vi "Read Theme.vi"(8 "error in":errorcluster, 11 "Theme in":refnum<class "Theme.lvclass">) -> (0 "error out":errorcluster, 1 "button colors":T2={"false color"={"border"=13816530, "fill"=16777215}, "hover color"={"border"=0, "fill"=0}, "press color"={"border"=1067897, "fill"=1067897}, "Boolean Text"=1668818, "Text.Font Name"="", "Text.Font Size"=0, "Bold?"=TRUE, "Itallic?"=FALSE}, 2 "dialog colors":T3={"Header"=1668818, "Background"=1668818, "Picture Background"=16777216}, 4 "message font":T1={"Text.Font Name"="Segoe UI", "Text.Font Size"=30, "Color"=0, "Text.Justification"=enum."Center", "messge color"={"border"=16777215, "fill"=16777215}}, 6 "input":T1={"Text.Font Name"="Segoe UI", "Text.Font Size"=30, "Color"=0, "Text.Justification"=enum."Center", "messge color"={"border"=16777215, "fill"=16777215}})   [LabVIEW 2021, in "Theme.lvclass"]
doc: "Read theme data from an object\n\n<b>Code Developed By:</b>\nTechnology Service Corporation\n1983 S Liberty Drive\nBloomington, IN 47403\nPhone: 812 558-7100\nwww.tsc.com/atcs\n\nDeveloper:\nDaniel Coons"
uses:
  Theme.lvclass
  Dialog colors--typedef.ctl
  Button colors--typedef.ctl
  message box--typdef.ctl
  Theme.lvclass/Theme.ctl
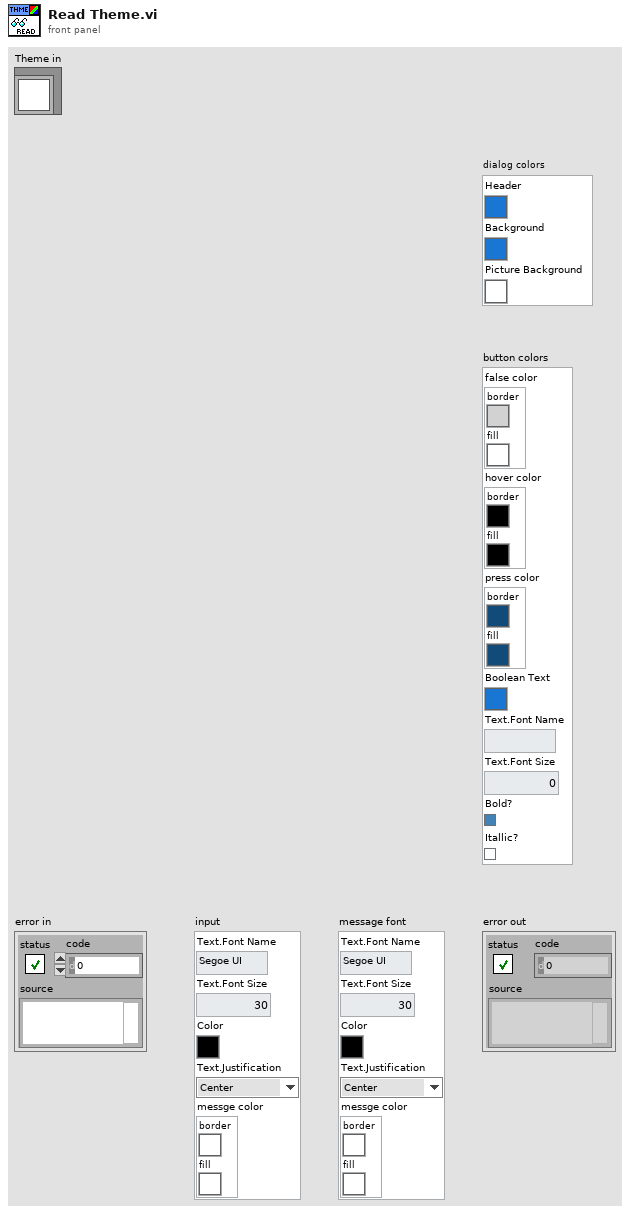
[diagram p1: front panel]
types:
  T1 = typedef "Theme.lvclass/message box--typdef.ctl" = cluster{"Text.Font Name":string, "Text.Font Size":u32, "Color":u32, "Text.Justification":enum16{"Left", "Center", "Right"}, "messge color":cluster{"border":u32, "fill":u32}}
  T2 = typedef "Theme.lvclass/Button colors--typedef.ctl" = cluster{"false color":cluster{"border":u32, "fill":u32}, "hover color":cluster{"border":u32, "fill":u32}, "press color":cluster{"border":u32, "fill":u32}, "Boolean Text":u32, "Text.Font Name":string, "Text.Font Size":u32, "Bold?":bool, "Itallic?":bool}
  T3 = typedef "Theme.lvclass/Dialog colors--typedef.ctl" = cluster{"Header":u32, "Background":u32, "Picture Background":u32}
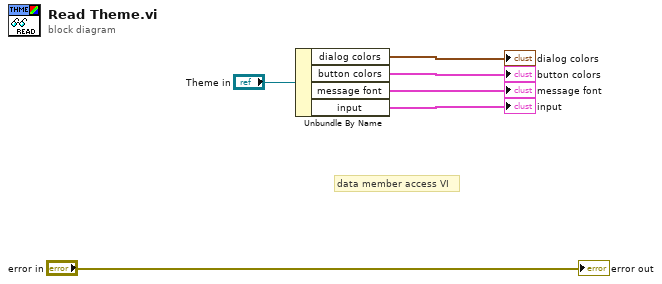
[diagram p0: block diagram]
diagram:
  # "data member access VI"
  n1 = Unbundle By Name("Theme in") -> ("dialog colors"=→"dialog colors":T3, "button colors"=→"button colors":T2, "message font"=→"message font":T1, "input"=→"input":T1)
  "error out" <- "error in"
